vi "read_settings.vi"(8 "error in":errorcluster) -> (0 "error out":errorcluster, 1 "Zone 3 PID":T1={"proportional gain (Kc)"=1.0, "integral time (Ti, min)"=0.01, "derivative time (Td, min)"=0.0} {"derivative time (Td, min)" format="%.3f"; "integral time (Ti, min)" format="%.3f"; "proportional gain (Kc)" format="%.3f"}, 2 "Zone 2 PID":T1={"proportional gain (Kc)"=1.0, "integral time (Ti, min)"=0.01, "derivative time (Td, min)"=0.0} {"derivative time (Td, min)" format="%.3f"; "integral time (Ti, min)" format="%.3f"; "proportional gain (Kc)" format="%.3f"}, 3 "Zone 1 PID":T1={"proportional gain (Kc)"=1.0, "integral time (Ti, min)"=0.01, "derivative time (Td, min)"=0.0} {"derivative time (Td, min)" format="%.3f"; "integral time (Ti, min)" format="%.3f"; "proportional gain (Kc)" format="%.3f"}, 4 "Zone 1 SP":dbl, 5 "Zone 3 SP":dbl, 6 "Notes":string, 7 "Zone 2 SP":dbl)   [LabVIEW 2020]
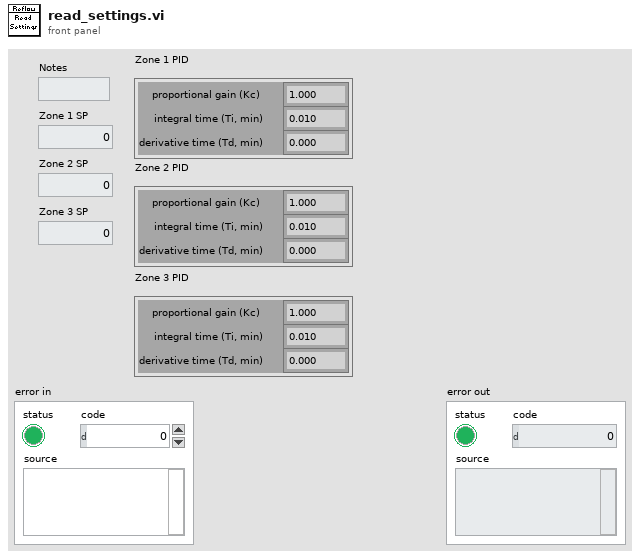
[diagram p1: front panel]
types:
  T1 = cluster{"proportional gain (Kc)":dbl, "integral time (Ti, min)":dbl, "derivative time (Td, min)":dbl}
  T2 = cluster{"Notes":string, "Zone 1 SP":dbl, "Zone 2 SP":dbl, "Zone 3 SP":dbl, "Zone 1 PID":cluster{"proportional gain (Kc)":dbl, "integral time (Ti, min)":dbl, "derivative time (Td, min)":dbl}, "Zone 2 PID":cluster{"proportional gain (Kc)":dbl, "integral time (Ti, min)":dbl, "derivative time (Td, min)":dbl}, "Zone 3 PID":cluster{"proportional gain (Kc)":dbl, "integral time (Ti, min)":dbl, "derivative time (Td, min)":dbl}}
  T3 = enum16{"open", "replace", "create", "open or create", "replace or create", "replace or create with confirmation"}
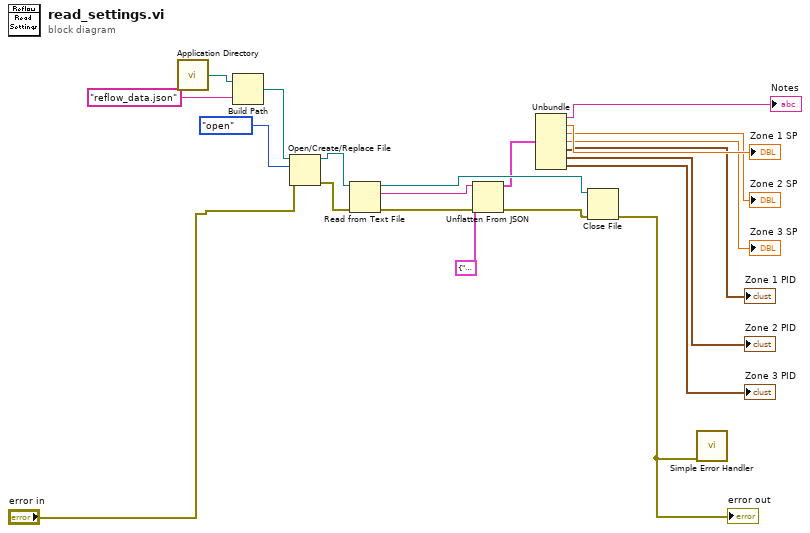
[diagram p0: block diagram]
diagram:
  n1 = call <vilib>:"Application Directory.vi"() -> ("Application Directory"=w20:path)
  n2 = Build Path(base path=w20, name or relative path="reflow_data.json") -> (appended path=w18:path)
  n3 = Open/Create/Replace File(file path (use dialog)=w18, error in="error in", operation (0:open)=T3."open") -> (refnum out=w17:refnum<file>, error out=w16:errorcluster)  [unwired: 3 in, 1 out]
  n4 = Read from Text File(file (use dialog)=w17, error in=w16) -> (refnum out=w14:refnum<file>, text=w11:string, error out=w1:errorcluster)  [unwired: 2 in, 1 out]
  n5 = Unflatten From JSON(JSON string=w11, type and defaults=T2 {"Notes"="", "Zone 1 SP"=0.0, "Zone 2 SP"=0.0, "Zone 3 SP"=0.0, "Zone 1 PID"={"proportional gain (Kc)"=0.0, "integral time (Ti, min)"=0.0, "derivative time (Td, min)"=0.0}, "Zone 2 PID"={"proportional gain (Kc)"=0.0, "integral time (Ti, min)"=0.0, "derivative time (Td, min)"=0.0}, "Zone 3 PID"={"proportional gain (Kc)"=0.0, "integral time (Ti, min)"=0.0, "derivative time (Td, min)"=0.0}} ("output cluster"), error in (no error)=w1) -> (value=w9:T2, error out=w15:errorcluster)  [unwired: 4 in]
  n6 = Unbundle(w9) -> ("Notes"=→"Notes":string, "Zone 1 SP"=→"Zone 1 SP":dbl, "Zone 2 SP"=→"Zone 2 SP":dbl, "Zone 3 SP"=→"Zone 3 SP":dbl, "Zone 1 PID"=→"Zone 1 PID":T1, "Zone 2 PID"=→"Zone 2 PID":T1, "Zone 3 PID"=→"Zone 3 PID":T1)
  n7 = Close File(refnum=w14, error in=w15) -> (error out=w12:errorcluster)  [unwired: 1 out]
  "error out" <- w12
  n8 = call <vilib>:"Simple Error Handler.vi"("error in (no error)"=w12) -> ()  [unwired: 4 in, 5 out]
